vi "temperatura_luminosidade_grafico_termometro.vi"() -> ()   [LabVIEW 2018]
uses:
  <vilib>/Instr/_visa.llb/VISA Configure Serial Port (Instr).vi
panel:
  in  "Arquivo":path
  out "Waveform Chart":cluster{i32, "number":i32}(graph)
  out "Thermometer":dbl(slide) scale=0.0..100.0
  in  "?":bool
  in  "VISA resource name":refnum<visa-resource-name>
  in  "?":bool
  out "?":bool
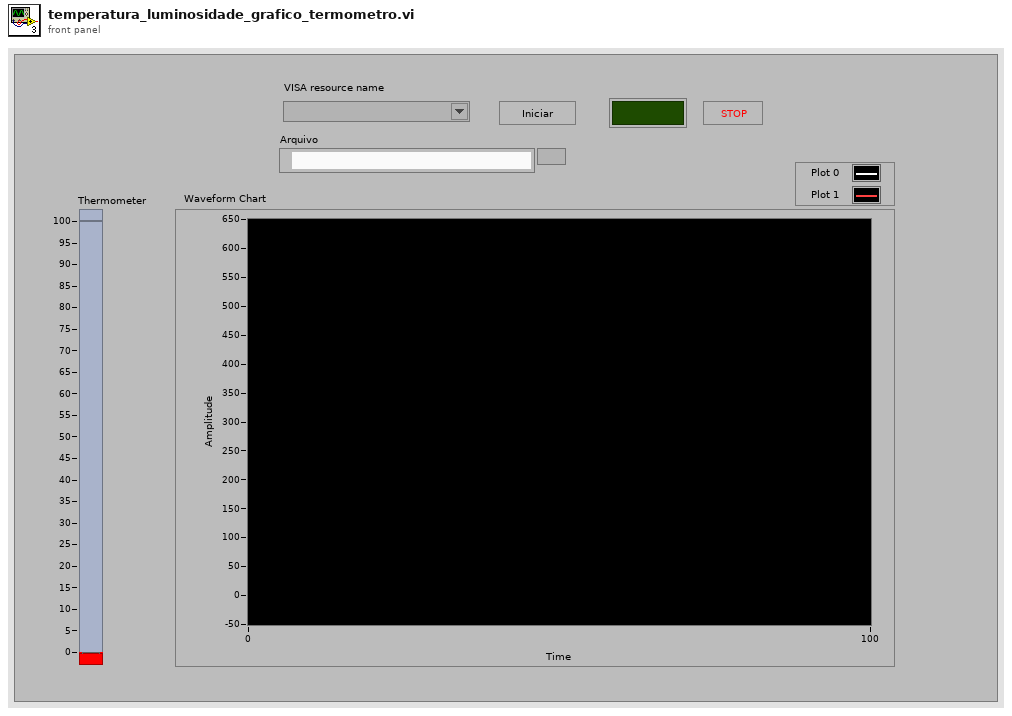
[diagram p1: front panel]
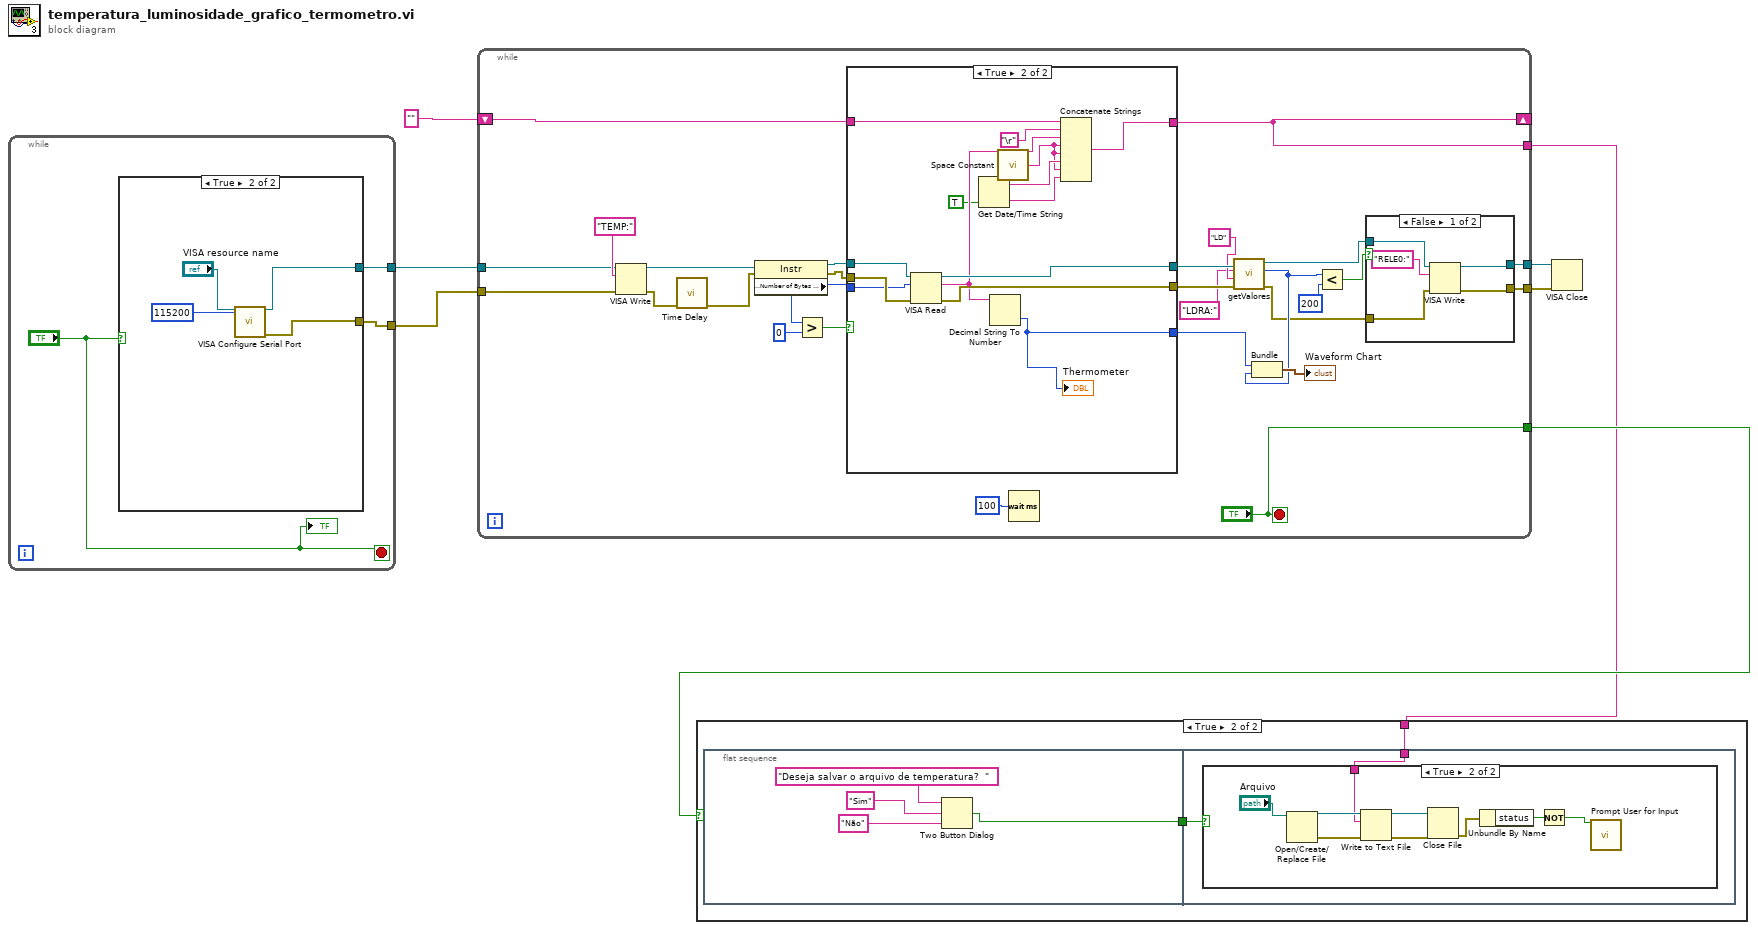
[diagram p0: block diagram]
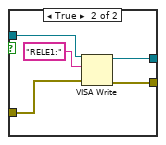
[diagram p4: hidden frame]
diagram:
  n1 = while {
    tunnel: [w9] -> w2
    tunnel: [w8] -> w1
    stop <- "?" stop-if-true
    n2 = case shown="True" "?" {
      tunnel: [_ w12] -> w9
      tunnel: [_ w11] -> w8
      frame False {
      }
      frame True {
        n3 = call-poly "VISA Configure Serial Port"("VISA resource name"="VISA resource name", "baud rate (9600)"=u32 115200) -> ("VISA resource name out"=w11:refnum<visa-resource-name>, "error out"=w12:errorcluster)  [unwired: 12 in]
      }
    }
    "?" <- "?"
  }
  n4 = while {
    shift-right: [w30] -> _
    shift-left: "" -> [w33]
    tunnel: ["?"] -> w6
    tunnel: [w30] -> w5
    tunnel: [w21] -> w4
    tunnel: [w20] -> w3
    tunnel: w2 -> [w16]
    tunnel: w1 -> [w15]
    stop <- "?" stop-if-true
    n5 = VISA Write(VISA resource name=w15, write buffer="TEMP:", error in (no error)=w16) -> (VISA resource name out=w40:refnum<visa-resource-name>, error out=w41:errorcluster)  [unwired: 1 out]
    n6 = call "Time Delay"("error in (no error)"=w41) -> ("error out"=w39:errorcluster)  [unwired: 10 in]
    n7 = property class="Instr"(reference=w40, error in=w39) -> (reference out=w36:refnum<visa-resource-name>, error out=w35:errorcluster, "Serial Settings:Number of Bytes at Serial Port"=w34:u32)
    n8 = Greater?(x=w34, y=u32 0) -> (0:w38:bool)
    n9 = case shown="True" w38 {
      tunnel: w36 -> [w55 w69]
      tunnel: w35 -> [w54 w68]
      tunnel: w34 -> [_ w67]
      tunnel: [w55 w66] -> w29
      tunnel: [w54 w65] -> w28
      tunnel: [w53 w57] -> w30
      tunnel: w33 -> [w53 w64]
      tunnel: [_ w56] -> w27
      frame False {
      }
      frame True {
        n10 = VISA Read(VISA resource name=w69, byte count=w67, error in (no error)=w68) -> (VISA resource name out=w66:refnum<visa-resource-name>, read buffer=w62:string, error out=w65:errorcluster)  [unwired: 1 out]
        n11 = Get Date/Time String(want seconds? (F)=TRUE) -> (date string=w61:string, time string=w59:string)  [unwired: 2 in]
        n12 = Decimal String To Number(string=w62) -> (number=w56:i32)  [unwired: 2 in, 1 out]
        "Thermometer" <- w56
        n13 = call <vilib>:"Space Constant.vi"() -> ("String"=w60:string)
        n14 = Concatenate Strings(w64, "\r", w62, w60, w60, w61, w60, w59) -> (w57:string)
      }
    }
    n15 = Wait (ms)(milliseconds to wait=u32 100) -> ()  [unwired: 1 out]
    n16 = call "getValores.vi"("error in (no error)"=w28, "verificação"="LD" ("enviar código"), "enviar código"="LDRA:", "VISA Refnum in"=w29) -> ("error out"=w17:errorcluster, "number"=w23:i32, "VISA Refnum out"=w18:refnum<visa-resource-name>)  [unwired: 5 in]
    n17 = Bundle(w27, "number"=w23) -> (→"Waveform Chart":cluster{i32, "number":i32})  [unwired: 1 in]
    n18 = Less?(x=w23, y=200) -> (x < y?=w19:bool)
    n19 = case shown="False" w19 {
      tunnel: [w43 w52] -> w21
      tunnel: [w44 w51] -> w20
      tunnel: w18 -> [w46 w49]
      tunnel: w17 -> [w45 w48]
      frame False {
        n20 = VISA Write(VISA resource name=w46, write buffer="RELE0:", error in (no error)=w45) -> (VISA resource name out=w43:refnum<visa-resource-name>, error out=w44:errorcluster)  [unwired: 1 out]
      }
      frame True {
        n21 = VISA Write(VISA resource name=w49, write buffer="RELE1:", error in (no error)=w48) -> (VISA resource name out=w52:refnum<visa-resource-name>, error out=w51:errorcluster)  [unwired: 1 out]
      }
    }
  }
  n22 = case shown="True" w6 {
    tunnel: w5 -> [_ w71]
    frame False {
    }
    frame True {
      n23 = flat-sequence {
        tunnel: [w72] -> w70
        tunnel: w71 -> [w77]
        tunnel: w70 -> [w76]
        frame #0 {
          n24 = Two Button Dialog(message="Deseja salvar o arquivo de temperatura?  ", 1:"Não" ("F button name (\"Cancel\")"), 2:"Sim" ("T button name (\"OK\")")) -> (T button?=w72:bool)
        }
        frame #1 {
          n25 = case shown="True" w76 {
            tunnel: w77 -> [_ w83]
            frame False {
            }
            frame True {
              n26 = Open/Create/Replace File(file path (use dialog)="Arquivo") -> (refnum out=w85:refnum<file>, error out=w84:errorcluster)  [unwired: 5 in, 1 out]
              n27 = Write to Text File(file (use dialog)=w85, text=w83, error in=w84) -> (refnum out=w82:refnum<file>, error out=w81:errorcluster)  [unwired: 1 in, 1 out]
              n28 = Close File(refnum=w82, error in=w81) -> (error out=w80:errorcluster)  [unwired: 1 out]
              n29 = Unbundle By Name(w80) -> ("status"=w79:bool)
              n30 = Not(x=w79) -> (.not. x?=w78:bool)
              n31 = call "Prompt User for Input"("Enable"=w78) -> ()  [unwired: 17 in, 2 out]
            }
          }
        }
      }
    }
  }
  n32 = VISA Close(VISA resource name=w4, error in (no error)=w3) -> ()  [unwired: 1 out]
